vi "Create Message Transport.vi"(7 "Transport Name":string, 8 "error in":errorcluster, 10 "Transport Payload type":refnum<class "IMessagePayload.lvclass">, 11 "QueueMessageTransport in":refnum<class "QueueMessageTransport.lvclass">) -> (0 "error out":errorcluster, 3 "QueueMessageTransport out":refnum<class "QueueMessageTransport.lvclass">)   [LabVIEW 2016, in "QueueMessageTransport.lvclass"]
uses:
  QueueMessageTransport.lvclass
  IMessagePayload/IMessagePayload.lvclass
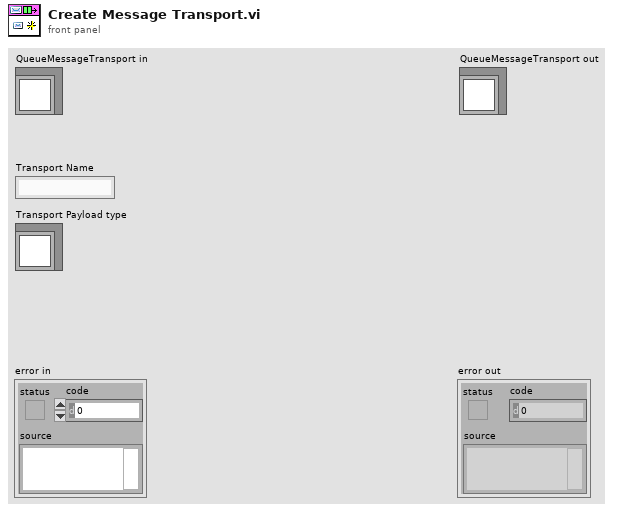
[diagram p1: front panel]
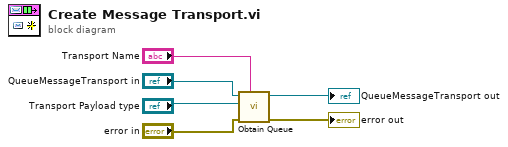
[diagram p0: block diagram]
diagram:
  n1 = call "Obtain Queue.vi"("Q Name"="Transport Name", "error in"="error in", "Q Element data type"="Transport Payload type", "QueueMessageTransport in"="QueueMessageTransport in") -> ("error out"=→"error out":errorcluster, "QueueMessageTransport out"=→"QueueMessageTransport out":refnum<class "QueueMessageTransport.lvclass">)  [unwired: 6 in]
